vi "Color Get Color Of Light Param.vi"(0 "a_data":dbl[](array[numeric]), 1 "a_Observer":u8, 5 "error in (no error)":errorcluster, 6 "a_CIEResolution":u8) -> (3 "function return":i16, 4 "error out":errorcluster, 7 "a_smally out":dbl, 10 "a_Colortemperature out":dbl, 11 "a_bigZ out":dbl, 12 "a_u out":dbl, 13 "a_v out":dbl, 14 "a_data out":dbl[](array[numeric]), 15 "a_bigY out":dbl, 17 "a_smallx out":dbl, 18 "a_smallz out":dbl, 19 "a_bigX out":dbl)   [LabVIEW 2013, in "AVSirrad.lvlib"]
doc: "DLL_API short int __stdcall Color_GetColorOfLightParam\n(\n DataType *a_data,\n unsigned char a_CIEResolution,\n unsigned char a_Observer,\n double *a_smallx,\n double *a_smally,\n double *a_smallz,\n double *a_bigX,\n double *a_bigY,\n double *a_bigZ,\n double *a_u,\n double *a_v,\n double *a_Colortemperature\n);"
uses:
  AVSirrad.lvlib
  AVSIRRAD/Examples/Labview/build/AVSirrad.dll
panel:
  in  "a_Colortemperature":dbl
  in  "a_v":dbl
  in  "a_u":dbl
  in  "a_bigZ":dbl
  in  "a_bigY":dbl
  in  "a_bigX":dbl
  in  "a_smallz":dbl
  in  "a_smally":dbl
  in  "a_smallx":dbl
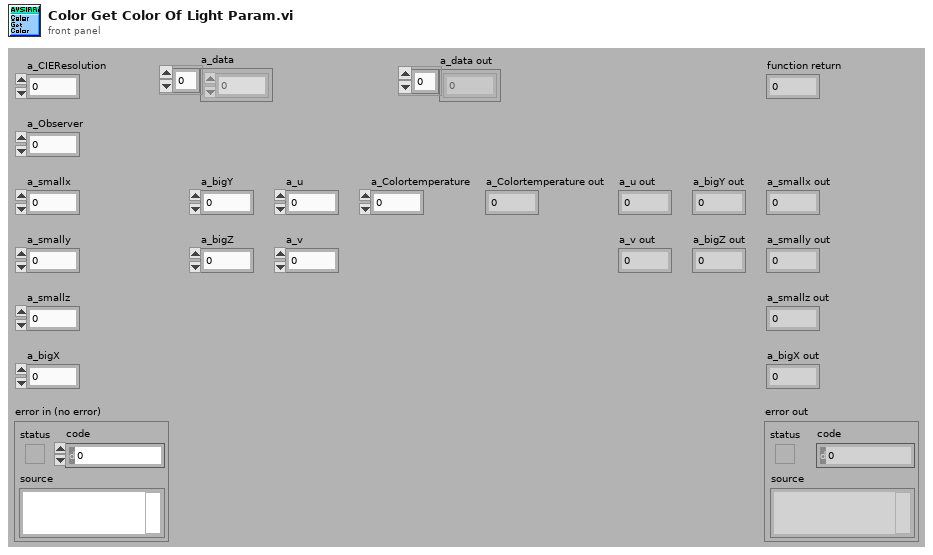
[diagram p1: front panel]
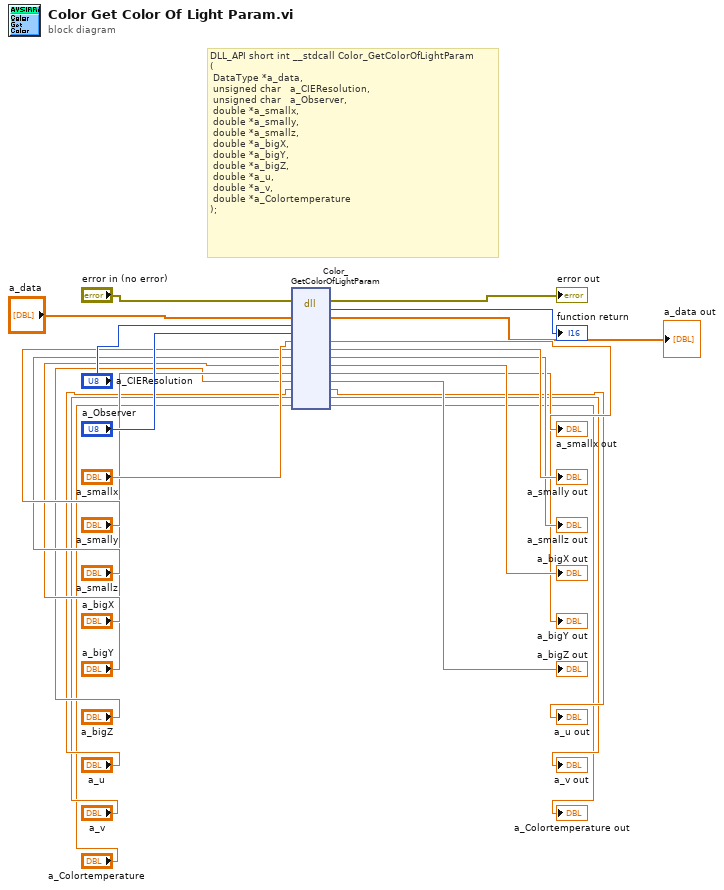
[diagram p0: block diagram]
diagram:
  # "DLL_API short int __stdcall Color_GetColorOfLightParam\n(\n\tDataType *a_data,\n\tunsigned char   a_CIEResolution,\n\tunsigned char   a_Observer,\n\tdouble *a_smallx,\n\tdouble *a_smally,\n\tdouble *a_smallz,\n\tdouble *a_bigX,\n\tdouble *a_bigY,\n\tdouble *a_bigZ,\n\tdouble *a_u,\n\tdouble *a_v,\n\tdouble *a_Colortemperature\n);"
  n1 = dll-call lib="C:/AVSIRRAD/Examples/Labview/build/AVSirrad.*" fn="Color_GetColorOfLightParam"(error in="error in (no error)", "a_data"="a_data", "a_CIEResolution"="a_CIEResolution", "a_Observer"="a_Observer", "a_smallx"="a_smallx", "a_smally"="a_smally", "a_smallz"="a_smallz", "a_bigX"="a_bigX", "a_bigY"="a_bigY", "a_bigZ"="a_bigZ", "a_u"="a_u", "a_v"="a_v", "a_Colortemperature"="a_Colortemperature") -> (error out=→"error out":errorcluster, "return type"=→"function return":i16, "a_data"=→"a_data out":dbl[], "a_smallx"=→"a_smallx out":dbl, "a_smally"=→"a_smally out":dbl, "a_smallz"=→"a_smallz out":dbl, "a_bigX"=→"a_bigX out":dbl, "a_bigY"=→"a_bigY out":dbl, "a_bigZ"=→"a_bigZ out":dbl, "a_u"=→"a_u out":dbl, "a_v"=→"a_v out":dbl, "a_Colortemperature"=→"a_Colortemperature out":dbl)  [unwired: 4 in, 1 out]
